vi "Robot_Orientation.vi"(2 "Sensor_Back":dbl, 3 "Distance_Sensor2Sensor":dbl, 4 "Sensor_Front":dbl) -> (0 "Angle":dbl, 1 "Distance":dbl)   [LabVIEW 2015]
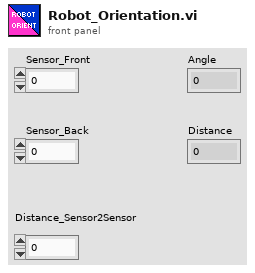
[diagram p1: front panel]
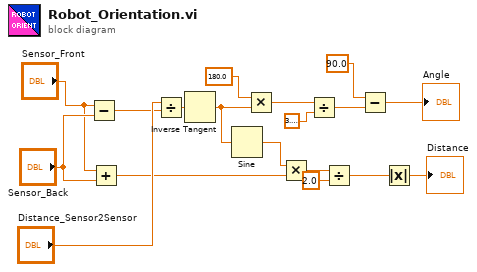
[diagram p0: block diagram]
diagram:
  n1 = Subtract(x="Sensor_Front", y="Sensor_Back") -> (x-y=w9:dbl)
  n2 = Add(x="Sensor_Front", y="Sensor_Back") -> (x+y=w10:dbl)
  n3 = Divide(x="Distance_Sensor2Sensor", y=w9) -> (x/y=w1:dbl)
  n4 = Inverse Tangent(1:w1) -> (0:w5:dbl)
  n5 = Sine(x=w5) -> (sin(x)=w2:dbl)
  n6 = Multiply(x=180.0, y=w5) -> (x*y=w17:dbl)
  n7 = Multiply(x=w2, y=w10) -> (x*y=w3:dbl)
  n8 = Divide(x=w17, y=3.141592653589793) -> (x/y=w6:dbl)
  n9 = Divide(x=w3, y=2.0) -> (x/y=w14:dbl)
  n10 = Subtract(x=90.0, y=w6) -> (x-y=→"Angle":dbl)
  n11 = Absolute Value(x=w14) -> (abs(x)=→"Distance":dbl)
